vi "Encoder Motor.vi"(6 "Count Type":dbl, 8 "Motor Refnum":string, 9 "Inversion":bool, 10 "CAN ID":dbl, 11 "Encoder Refnum":string) -> ()   [LabVIEW 2018]
uses:
  <vilib>/Rock Robotics/WPI/ThirdParty/Phoenix-LabVIEW/Motor Controller/Controls/CTRE_Phoenix_MotorControl_NeutralMode.ctl
  <vilib>/Rock Robotics/WPI/ThirdParty/Phoenix-LabVIEW/Motor Controller/Controls/CTRE_Phoenix_MotorControl_FeedbackDevice.ctl
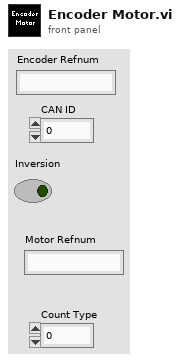
[diagram p1: front panel]
types:
  T1 = typedef "CTRE_Phoenix_MotorControl_FeedbackDevice.ctl" = i8
  T2 = typedef "CTRE_Phoenix_MotorControl_NeutralMode.ctl" = enum8{"EEPROMSetting", "Override to Coast", "Override to Brake"}
  T3 = typedef "WPI_MotorControlDeviceRef.ctl" = cluster{"DeviceStatus":errorcluster, "Type":T4, "PWM":cluster{"PWM Channel":T5, "DeadBand":T6}, "CAN":cluster{"Device Number":u8, "SetOutput VI Ref":variant, "GetOutput VI Ref":variant, "Enable VI Ref":variant, "Disable VI Ref":variant, "Data":variant}, "Invert":bool, "DIO PWM":cluster{"PWM \"Enable\" Channel":T5, "DIOChannel":T7, "PWM Rate":dbl}}
  T4 = typedef "WPI_MotorControlType.ctl" = enum16{"PWM", "CAN", "DIO PWM"}
  T5 = typedef "FPGA_DIOPWMChannel.ctl" = enum8{"PWM 0", "PWM 1", "PWM 2", "PWM 3", "PWM 4", "PWM 5", "PWM 6", "PWM 7", "PWM 8", "PWM 9", "PWM MXP 0", "PWM MXP 1", "PWM MXP 2", "PWM MXP 3", "PWM MXP 4", "PWM MXP 5", "PWM MXP 6", "PWM MXP 7", "PWM MXP 8", "PWM MXP 9", "Invalid"}
  T6 = typedef "WPI_PWMDeadband.ctl" = cluster{"Name":string, "maxPositivePwm":i32, "minPositivePwm":i32, "centerPwm":i32, "maxNegativePwm":i32, "minNegativePwm":i32, "angularRange":u16}
  T7 = typedef "FPGA_DIOChannel.ctl" = enum8{"DIO 0", "DIO 1", "DIO 2", "DIO 3", "DIO 4", "DIO 5", "DIO 6", "DIO 7", "DIO 8", "DIO 9", "DIO MXP 0", "DIO MXP 1", "DIO MXP 2", "DIO MXP 3", "DIO MXP 4", "DIO MXP 5", "DIO MXP 6", "DIO MXP 7", "DIO MXP 8", "DIO MXP 9", "DIO MXP 10", "DIO MXP 11", "DIO MXP 12", "DIO MXP 13", "DIO MXP 14", "DIO MXP 15", "SPI Port CS1", "SPI Port CS2", "SPI Port CS3", "SPI Port MISO", "SPI Port MOSI", "Invalid"}
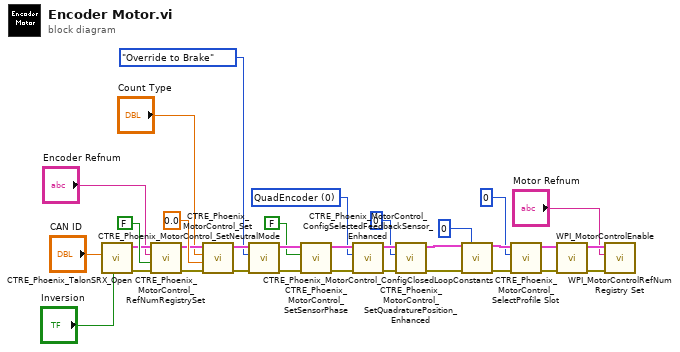
[diagram p0: block diagram]
diagram:
  w23 = T1 0 items=["None"=-1, "QuadEncoder"=0, "Analog"=2, "Tachometer"=4, "Pulse Width Encoded Position"=8, "Sensor Sum (S0 + S1)"=9, "Sensor Difference (D0 - D1)"=10, "Remote Source 0"=11, "Remote Source 1"=12, "Software Emulated"=15] ("Feedback Device")
  n1 = call <vilib>:"CTRE_Phoenix_TalonSRX_Open.vi"("Invert"="Inversion", "Device Number"="CAN ID") -> ("error out"=w8:errorcluster, "CAN Talon SRX Ref"=w9:T3)  [unwired: 8 in]
  n2 = call <vilib>:"CTRE_Phoenix_MotorControl_RefNumRegistrySet.vi"("error in (no error)"=w8, "Test Mode Only"=FALSE, "refnum name"="Encoder Refnum", "PhoenixMotorControlDevRef"=w9) -> ("error out"=w6:errorcluster, "PhoenixMotorControlDevRef"=w7:T3)  [unwired: 6 in]
  n3 = call <vilib>:"CTRE_Phoenix_MotorControl_Set.vi"("error in (no error)"=w6, "Output"=0.0, "Control Mode"="Count Type", "PhoenixMotorControlDevRef"=w7) -> ("error out"=w27:errorcluster, "PhoenixMotorControlDevRef"=w31:T3)  [unwired: 6 in]
  n4 = call <vilib>:"CTRE_Phoenix_MotorControl_SetNeutralMode.vi"("error in (no error)"=w27, "Motor Control Neutral Mode"=CTRE_Phoenix_MotorControl_NeutralMode."Override to Brake", "PhoenixMotorControlDevRef"=w31) -> ("error out"=w29:errorcluster, "PhoenixMotorControlDevRef"=w28:T3)  [unwired: 7 in]
  n5 = call <vilib>:"CTRE_Phoenix_MotorControl_SetSensorPhase.vi"("error in (no error)"=w29, "PhaseSensor"=FALSE, "PhoenixMotorControlDevRef"=w28) -> ("error out"=w25:errorcluster, "PhoenixMotorControlDevRef"=w24:T3)  [unwired: 7 in]
  n6 = call <vilib>:"CTRE_Phoenix_MotorControl_ConfigSelectedFeedbackSensor_Enhanced.vi"("error in (no error)"=w25, "Feedback Device"=w23, "PhoenixMotorControlDevRef"=w24) -> ("error out"=w21:errorcluster, "PhoenixMotorControlDevRef"=w22:T3)  [unwired: 7 in]
  n7 = call <vilib>:"CTRE_Phoenix_MotorControl_SetQuadraturePosition_Enhanced.vi"("error in (no error)"=w21, "New Position"=0, "PhoenixMotorControlDevRef"=w22) -> ("error out"=w18:errorcluster, "PhoenixMotorControlDevRef"=w19:T3)  [unwired: 7 in]
  n8 = call <vilib>:"CTRE_Phoenix_MotorControl_ConfigClosedLoopConstants.vi"("PhoenixMotorControlDevRef"=w19, "slotIdx"=0, "error in (no error)"=w18) -> ("PhoenixMotorControlDevRef"=w15:T3, "error out"=w16:errorcluster)  [unwired: 11 in]
  n9 = call <vilib>:"CTRE_Phoenix_MotorControl_SelectProfile Slot.vi"("error in (no error)"=w16, "slotIdx"=0, "PhoenixMotorControlDevRef"=w15) -> ("error out"=w11:errorcluster, "PhoenixMotorControlDevRef"=w12:T3)  [unwired: 7 in]
  n10 = call <vilib>:"WPI_MotorControlEnable.vi"("error in (no error)"=w11, "CAN MotorDevRef"=w12) -> ("error out"=w33:errorcluster, "CAN MotorDevRef"=w32:T3)  [unwired: 8 in]
  n11 = call <vilib>:"WPI_MotorControlRefNum Registry Set.vi"("error in (no error)"=w33, "refnum name"="Motor Refnum", "MotorControlDevRef"=w32) -> ()  [unwired: 7 in, 2 out]
